vi "ABR3-Set Level Order.vi"(0 "Runtime In":T1={"Ceiling"=0.0, "Threshold"=0.0, "Crossed?"=FALSE, "Step"=0, "Stop"=0, "Avgs"=0, "Level"=0.0, "AI Npts"=0, "Doubled?"=FALSE, "Gain"=0.0, "NWindowPts"=0, "dt"=0.0, "Cal"=path "", "Freq"=0.0, "AO Channels"=[], "AltPol"=FALSE, "AO Npts"=0, "AO Fs"=0.0, "Start"=0, "Stop max"=0, "Ear"=enum."Right", "Waveform"=enum."TONE PIP", "RepRate"=0.0, "CAP or ABR"=1, "LMasker"=0.0, "SeqVar"=enum."Signal Level", "Reps/buffer"=0, "Avg Mode"=enum."Neural/CM", "Wav"=path "", "Order"=enum."Sequential", "Levels"=[], "ControlVal"=0.0, "innerIndex"=0, "indexStep"=0} {"CAP or ABR" items=["CAP", "ABR"]}, 7 "Controls":T5) -> (4 "Runtime Out":T1={"Ceiling"=0.0, "Threshold"=0.0, "Crossed?"=FALSE, "Step"=0, "Stop"=0, "Avgs"=0, "Level"=0.0, "AI Npts"=0, "Doubled?"=FALSE, "Gain"=0.0, "NWindowPts"=0, "dt"=0.0, "Cal"=path "", "Freq"=0.0, "AO Channels"=[], "AltPol"=FALSE, "AO Npts"=0, "AO Fs"=0.0, "Start"=0, "Stop max"=0, "Ear"=enum."Right", "Waveform"=enum."TONE PIP", "RepRate"=0.0, "CAP or ABR"=1, "LMasker"=0.0, "SeqVar"=enum."Signal Level", "Reps/buffer"=0, "Avg Mode"=enum."Neural/CM", "Wav"=path "", "Order"=enum."Sequential", "Levels"=[], "ControlVal"=0.0, "innerIndex"=0, "indexStep"=0} {"CAP or ABR" items=["CAP", "ABR"]})   [LabVIEW 2020]
uses:
  TypeDefs/ABR3-Runtime Data.ctl
  epl-vi-lib/Utility VIs/Type Defs/Left-Right ring.ctl
  TypeDefs/ABR-Waveform Enum.ctl
  TypeDefs/ABR3-Seq Var Enum.ctl
  TypeDefs/ABR3-Controls.ctl
  epl-vi-lib/Utility VIs/Math VIs/LinSpace (start-stop-step).vi
  <vilib>/Analysis/1siggen.llb/Riffle Array (DBL).vi
  <vilib>/Analysis/NI_AALBase.lvlib
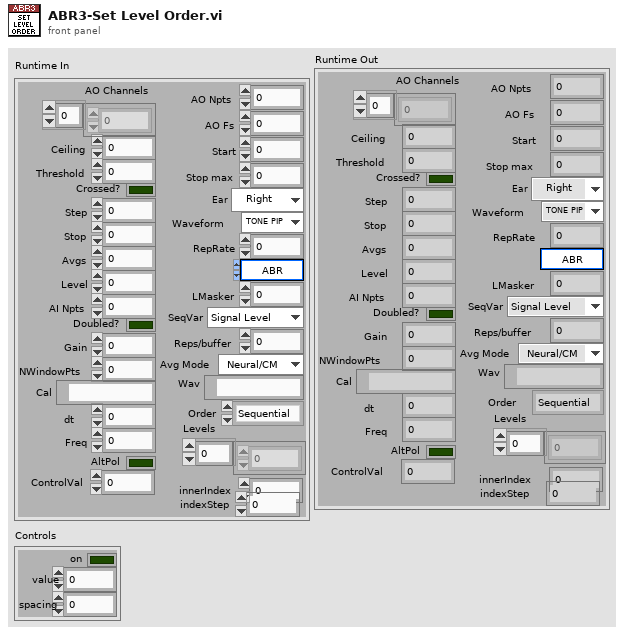
[diagram p1: front panel]
types:
  T1 = typedef "ABR3-Runtime Data.ctl" = cluster{"Ceiling":dbl, "Threshold":dbl, "Crossed?":bool, "Step":i32, "Stop":i32, "Avgs":i32, "Level":dbl, "AI Npts":i32, "Doubled?":bool, "Gain":dbl, "NWindowPts":i32, "dt":dbl, "Cal":path, "Freq":dbl, "AO Channels":i32[], "AltPol":bool, "AO Npts":i32, "AO Fs":dbl, "Start":i32, "Stop max":i32, "Ear":T2, "Waveform":T3, "RepRate":dbl, "CAP or ABR":u16, "LMasker":dbl, "SeqVar":T4, "Reps/buffer":i32, "Avg Mode":enum16{"Neural/CM", "ANOW"}, "Wav":path, "Order":enum16{"Sequential", "Random"}, "Levels":dbl[], "ControlVal":dbl, "innerIndex":i32, "indexStep":i32}
  T2 = typedef "Left-Right ring.ctl" = enum16{"Right", "Left"}
  T3 = typedef "ABR-Waveform Enum.ctl" = enum16{"TONE PIP", "CLICK", "FILE", "CHIRP", "NOISE", "VERHULST"}
  T4 = typedef "ABR3-Seq Var Enum.ctl" = enum16{"Signal Level", "Masker Level"}
  T5 = typedef "ABR3-Controls.ctl" = cluster{"on":bool, "value":dbl, "spacing":i32}
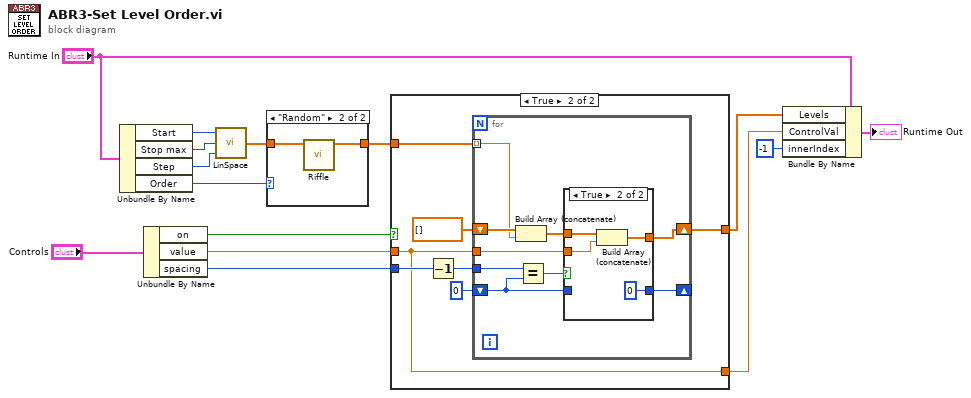
[diagram p0: block diagram]
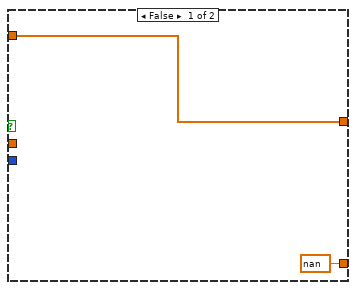
[diagram p2: hidden frame]
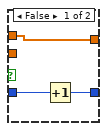
[diagram p3: hidden frame]
diagram:
  n1 = Unbundle By Name("Runtime In") -> ("Start"=w13:i32, "Stop max"=w12:i32, "Step"=w11:i32, "Order"=w10:enum16{"Sequential", "Random"})
  n2 = Unbundle By Name("Controls") -> ("on"=w9:bool, "value"=w8:dbl, "spacing"=w7:i32)
  n3 = call-poly "LinSpace.vi"("Step"=w11, "Stop"=w12, "Start"=w13) -> ("Array"=w14:dbl[])  [unwired: 1 in, 1 out]
  n4 = case shown="\"Random\"" w10 {
    tunnel: w14 -> [w16 w18]
    tunnel: [w16 w17] -> w15
    frame "Sequential", Default {
    }
    frame "Random" {
      n5 = call-poly <vilib>:"Riffle.vi"("X"=w18) -> ("Riffled {X}"=w17:dbl[])  [unwired: 8 in, 2 out]
    }
  }
  n6 = case shown="True" w9 {
    tunnel: w15 -> [w20 w24]
    tunnel: w8 -> [_ w21]
    tunnel: w7 -> [_ w23]
    tunnel: [w20 w22] -> w4
    tunnel: [nan ("value") w21] -> w3
    frame False {
    }
    frame True {
      n7 = Decrement(x=w23) -> (x-1=w27:i32)
      n8 = for {
        tunnel: w24 -> [w33] mode=indexing
        tunnel: w21 -> [w31]
        tunnel: w27 -> [w36]
        shift-right: [w29] -> _
        shift-left: 0 -> [w28]
        shift-right: [w30] -> w22
        shift-left: dbl[] [] ("Array") -> [w34]
        n9 = Build Array (concatenate)(w34, w33) -> (w32:dbl[])
        n10 = Equal?(x=w36, y=w28) -> (x = y?=w35:bool)
        n11 = case shown="True" w35 {
          tunnel: w32 -> [w37 w43]
          tunnel: w31 -> [_ w42]
          tunnel: [w37 w41] -> w30
          tunnel: [w38 0] -> w29
          tunnel: w28 -> [w39 _]
          frame False {
            n12 = Increment(x=w39) -> (x+1=w38:i32)
          }
          frame True {
            n13 = Build Array (concatenate)(w43, w42) -> (w41:dbl[])
          }
        }
      }
    }
  }
  n14 = Bundle By Name(cluster="Runtime In", "Levels"=w4, "ControlVal"=w3, "innerIndex"=-1) -> (→"Runtime Out":T1)
